vi "Pre Launch Init.vi"(11 "Example Actor in":refnum<class "Example Actor.lvclass">) -> (0 "error out":errorcluster, 3 "Example Actor out":refnum<class "Example Actor.lvclass">)   [LabVIEW 2016, in "Example Actor.lvclass"]
doc: "(<B>Filename</B>: Actor Framework.lvlib:Actor.lvclass:Pre Launch Init.vi)\n\nDefines behavior that occurs after the Launch Nested Actor method is invoked but before the actor's Actor Core method begins running.\n\nBy default, this method does nothing. A descendant class may override it to define behavior.\n\n--\nCopyright © 2017 Composed SystemsI All rights reserved.\n\nAuthor: Jon McBee <jon.mcbee@composed.io>\n\nThis library is provided \"AS IS\" ,WITHOUT WARRANTIES OR\nCONDITIONS OF ANY KIND, either express or implied.\n\nComposed Systems -- composed.io\n\nStream 0.0.1.1\nJon McBee - Composed Systems\nCopyright (c) 2017, Composed Systems"
uses:
  <userlib>/Composed Systems/Stream/Mediator/Example/Example Actor/Example Actor.lvclass
  C:/Program Files (x86)/National Instruments/LabVIEW 2016/vi.lib/ActorFramework/Actor/Actor.lvclass
  <vilib>/ActorFramework/Actor/Actor.lvclass/Actor.ctl
  <vilib>/ActorFramework/Message Enqueuer/Message Enqueuer.lvclass/Message Enqueuer.ctl
  <userlib>/Composed Systems/Stream/Mediator/Example/Example Actor/Example Actor.lvclass/Example Actor.ctl
  <userlib>/Composed Systems/Stream/Mediator/Example/Example Actor Messages/Sample Actor Data Msg/Sample Actor Data Msg.lvclass
  C:/Program Files (x86)/National Instruments/LabVIEW 2016/user.lib/Composed Systems/Stream/Mediator/Classes/Message AF Mediator/Message AF Mediator.lvclass
  <vilib>/ActorFramework/Message Enqueuer/Init from Existing Queue.vi
  <userlib>/Composed Systems/Stream/Mediator/Classes/Message Transport Actor Framework/Message Transport Actor Framework.lvclass
  C:/Program Files (x86)/National Instruments/LabVIEW 2016/user.lib/Composed Systems/Stream/Mediator/Classes/Message Transport Interface/Message Transport Interface.lvclass
  <vilib>/ActorFramework/Actor/Actor.lvclass
  <userlib>/Composed Systems/Stream/Mediator/Classes/Message Broker Interface Ref/Message Broker Interface Ref.lvclass
  <vilib>/ActorFramework/Message Enqueuer/Message Enqueuer.lvclass
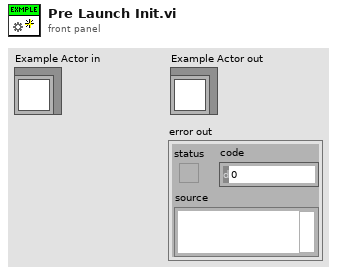
[diagram p1: front panel]
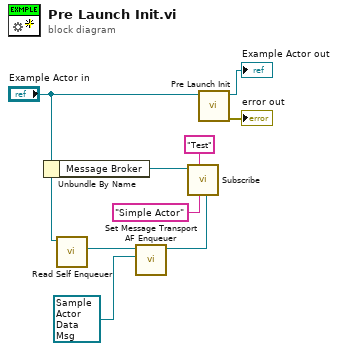
[diagram p0: block diagram]
diagram:
  n1 = Unbundle By Name("Example Actor in") -> ("Message Broker"=w6:refnum<class "Message Broker Interface Ref.lvclass">)
  n2 = call <vilib>:"Read Self Enqueuer.vi"("Actor"="Example Actor in") -> ("Self Enqueuer"=w4:refnum<class "Message Enqueuer.lvclass">)  [unwired: 10 in]
  n3 = call <userlib>:"Set Message Transport AF Enqueuer.vi"("Message AF Mediator"=refnum<class "Sample Actor Data Msg.lvclass"> refnum ("Sample Actor Data Msg.lvclass"), "Actor's Enqueuer"=w4) -> ("Message Transport Actor Framework out"=w3:refnum<class "Message Transport Actor Framework.lvclass">)  [unwired: 8 in, 1 out]
  n4 = call-dynamic "Subscribe.vi"("Message Transport Interface"=w3, "Subscriber Name"="Simple Actor", "Topic Name"="Test", "Message Broker Interface TAP in"=w6) -> ()  [unwired: 5 in, 3 out]
  n5 = call-parent "Pre Launch Init.vi"("Actor in"="Example Actor in") -> ("error out"=→"error out":errorcluster, "Actor out"=→"Example Actor out":refnum<class "Example Actor.lvclass">)  [unwired: 9 in]
